vi "3a.vi"() -> ()   [LabVIEW 2015]
panel:
  out "Waveform Graph 3":dbl[](graph)
  out "Waveform Graph 2":dbl[](graph)
  out "Waveform Graph":dbl[](graph)
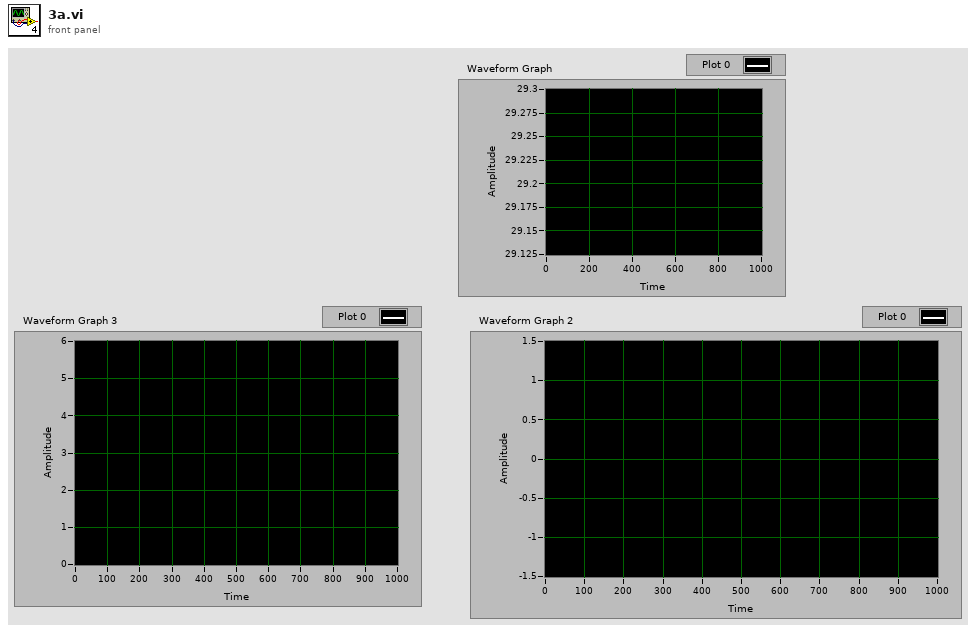
[diagram p1: front panel]
types:
  T1 = enum16{"open", "replace", "create", "open or create", "replace or create", "replace or create with confirmation"}
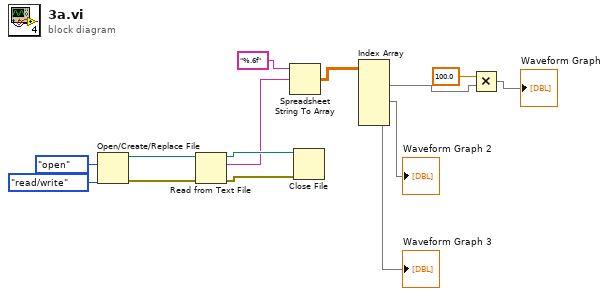
[diagram p0: block diagram]
diagram:
  n1 = Open/Create/Replace File(operation (0:open)=T1."open", access (0:read/write)=enum16{"read/write", "read-only", "write-only"}."read/write") -> (refnum out=w10:refnum<file>, error out=w12:errorcluster)  [unwired: 4 in, 1 out]
  n2 = Read from Text File(file (use dialog)=w10, error in=w12) -> (refnum out=w9:refnum<file>, text=w5:string, error out=w11:errorcluster)  [unwired: 2 in, 1 out]
  n3 = Spreadsheet String To Array(format string="%.6f", spreadsheet string=w5) -> (array=w8:dbl[][])  [unwired: 2 in]
  n4 = Close File(refnum=w9, error in=w11) -> ()  [unwired: 2 out]
  n5 = Index Array(array=w8) -> (element #1=w2:dbl[], element #2=→"Waveform Graph 2":dbl[], element #3=→"Waveform Graph 3":dbl[])  [unwired: 6 in]
  n6 = Multiply(x=100.0, y=w2) -> (x*y=→"Waveform Graph":dbl[])
